vi "DAQ_Dyn Dig Meas Configure and Measure.vi"(0 "DAQmx Task In":refnum<k21>, 2 "Execution Option":T4, 5 "Timing and Trigger Settings":T1={"Timing Settings"={"Sample Clock Source"="OnboardClock", "Sample Rate (Hz)"=10000.0, "Number of Samples"=1000, "Active Edge"=10280}, "Trigger Settings"={"Trigger Type"=enum."No Trigger", "Digital Start Trigger Source"="", "Digital Start Trigger Edge"=10280}} {"Trigger Settings"."Digital Start Trigger Edge" items=["Rising"=10280, "Falling"=10171]; "Timing Settings"."Active Edge" items=["Rising"=10280, "Falling"=10171]; "Timing Settings"."Number of Samples" format="%.0p"; "Timing Settings"."Sample Rate (Hz)" format="%#_6p"}, 11 "error in":errorcluster) -> (4 "DAQmx Task Out":refnum<k21>, 6 "Measured Digital Patterns":digitalwaveform(graph), 8 "Port Digital Data":u32[](array[numeric]), 10 "Acquisition Time (s)":dbl format="%#.2p", 15 "error out":errorcluster)   [LabVIEW 2021, in "DAQ_Dynamic Digital Pattern Measurement.lvlib"]
doc: "Configure, initiate and fetch dynamic digital pattern measurements from the channels configured."
uses:
  DAQ_Dynamic Digital Pattern Measurement.lvlib
  Typedefs/Timing & Trigger Settings.ctl
  Typedefs/Timing Settings.ctl
  Typedefs/Trigger Settings.ctl
  Common/Typedefs/Execution Options - Measure.ctl
  <vilib>/DAQmx/read.llb/DAQmx Read (Digital 1D Wfm NChan NSamp).vi
  <vilib>/DAQmx/configure/timing.llb/DAQmx Timing (Sample Clock).vi
  <vilib>/DAQmx/configure/trigger.llb/DAQmx Start Trigger (Digital Edge).vi
  <vilib>/DAQmx/miscellaneous.llb/DAQmx Fill In Error Info.vi
  <resource>/objmgr/daqmx.rc
panel:
  # "Outputs"
  # "Inputs"
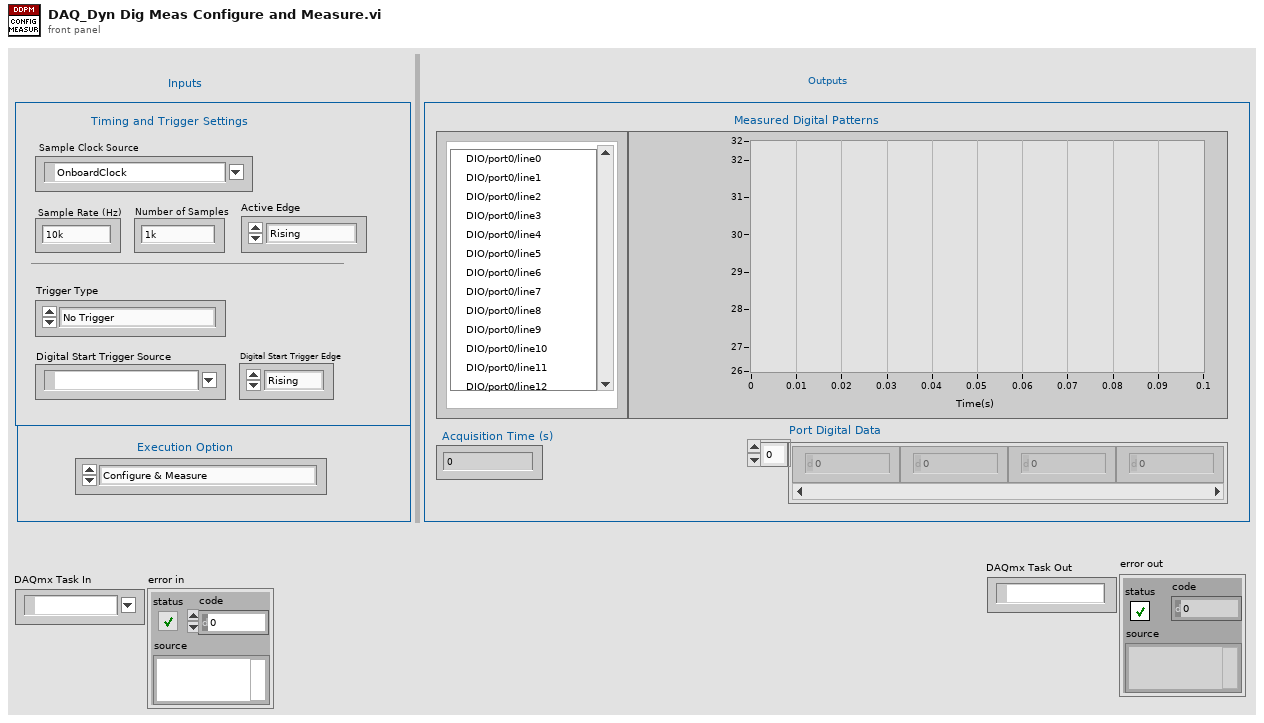
[diagram p1: front panel]
types:
  T1 = typedef "DAQ_Dynamic Digital Pattern Measurement.lvlib/Timing & Trigger Settings.ctl" = cluster{"Timing Settings":T2, "Trigger Settings":T3}
  T2 = typedef "DAQ_Dynamic Digital Pattern Measurement.lvlib/Timing Settings.ctl" = cluster{"Sample Clock Source":tag, "Sample Rate (Hz)":dbl, "Number of Samples":i32, "Active Edge":i32}
  T3 = typedef "DAQ_Dynamic Digital Pattern Measurement.lvlib/Trigger Settings.ctl" = cluster{"Trigger Type":enum16{"No Trigger", "Digital Start"}, "Digital Start Trigger Source":tag, "Digital Start Trigger Edge":i32}
  T4 = typedef "Execution Options - Measure.ctl" = enum16{"Configure & Measure", "Configure only", "Measure only"}
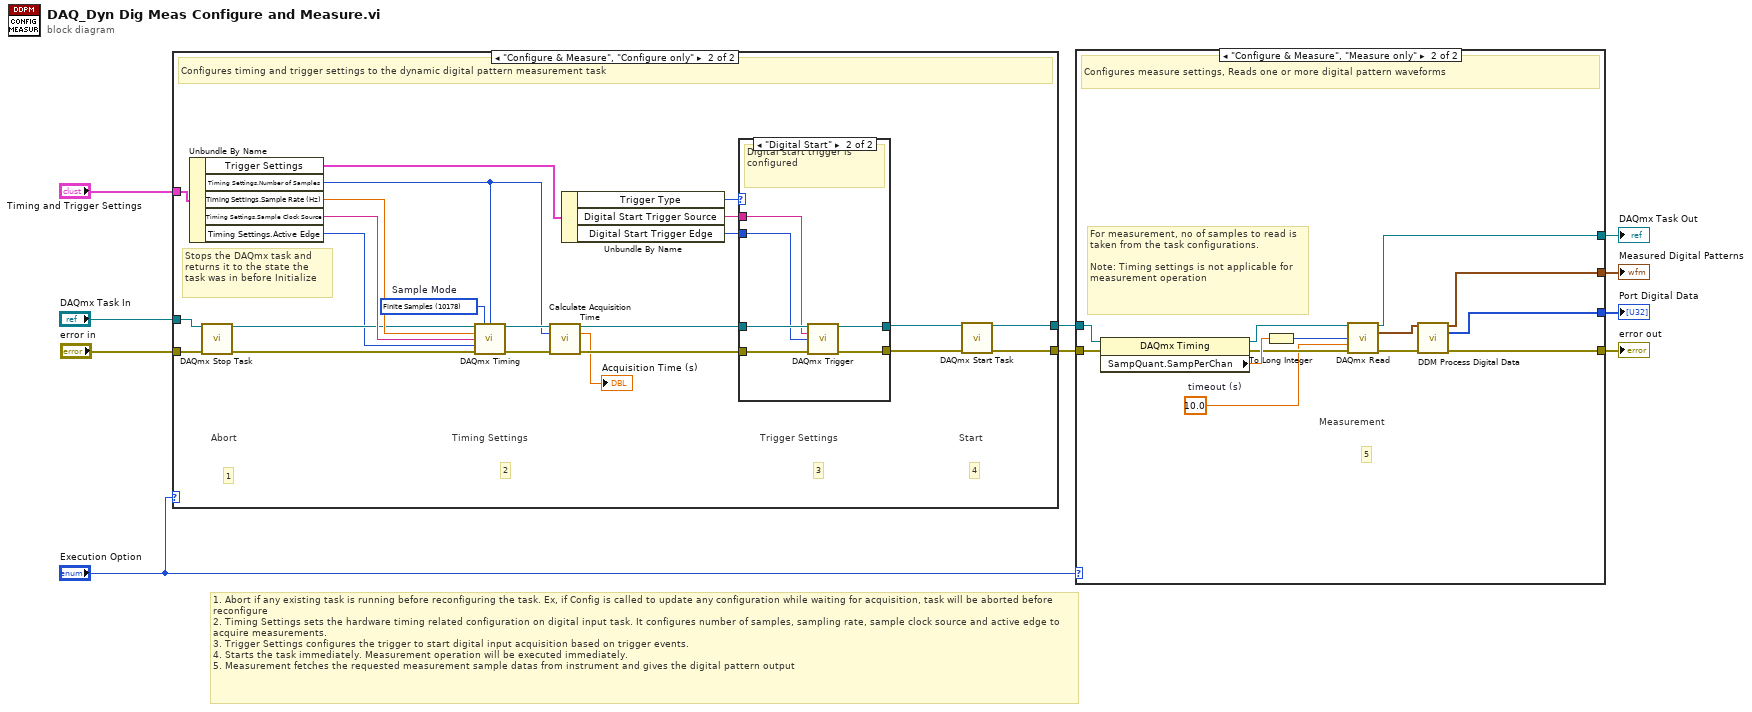
[diagram p0: block diagram]
diagram:
  # "1. Abort if any existing task is running before reconfiguring the task. Ex, if Config is called to update any configuration while waiting for acquisition, task will be aborted before reconfigure\n2. Timing Settings sets the hardware timing related configuration on digital input task. It configures number of samples, sampling rate, sample clock source and active edge to acquire measurements.\n3. Trigger Settings configures the trigger to start digital input acquisition based on trigger events.\n4. Starts the task immediately. Measurement operation will be executed immediately.\n5. Measurement fetches the requested measurement sample datas from instrument and gives the digital pattern output"
  n1 = case shown="\"Configure & Measure\", \"Configure only\"" "Execution Option" {
    tunnel: "error in" -> [w12 w18]
    tunnel: "DAQmx Task In" -> [w11 w20]
    tunnel: "Timing and Trigger Settings" -> [_ w30]
    tunnel: [w11 w16] -> w9
    tunnel: [w12 w27] -> w10
    frame Default {
      # "Skips Configurations (Channel, Timing and Trigger Settings)"
    }
    frame "Configure & Measure", "Configure only" {
      w14 = 10178 items=["Finite Samples"=10178, "Continuous Samples"=10123, "Hardware Timed Single Point"=12522]  # Sample Mode
      # "Stops the DAQmx task and returns it to the state the task was in before Initialize"
      # "4"
      # "Start"
      # "1"
      # "Abort"
      # "3"
      # "2"
      # "Trigger Settings"
      # "Timing Settings"
      # "Configures timing and trigger settings to the dynamic digital pattern measurement task"
      n2 = Unbundle By Name(w30) -> ("Trigger Settings"=w21:T3, "Timing Settings.Number of Samples"=w26:i32, "Timing Settings.Sample Rate (Hz)"=w31:dbl, "Timing Settings.Sample Clock Source"=w32:tag, "Timing Settings.Active Edge"=w13:i32)
      n3 = call <vilib>:"DAQmx Stop Task.vi"("task/channels in"=w20, "error in"=w18) -> ("task out"=w15:refnum<k21>, "error out"=w19:errorcluster)  [unwired: 12 in]
      n4 = call-poly <vilib>:"DAQmx Timing.vi"("task/channels in"=w15, "sample mode"=w14, "samples per channel"=w26, "rate"=w31, "source"=w32, "active edge"=w13, "error in"=w19) -> ("task out"=w35:refnum<k21>, "error out"=w34:errorcluster)  [unwired: 7 in]
      n5 = call "Calculate Acquisition Time.vi"("Refnum in"=w35, "Number of Samples"=w26, "error in (no error)"=w34) -> ("Refnum out"=w28:refnum<k21>, "Acquisition Time Period (s)"=→"Acquisition Time (s)":dbl, "error out"=w33:errorcluster)  [unwired: 10 in]
      n6 = Unbundle By Name(w21) -> ("Trigger Type"=w22:enum16{"No Trigger", "Digital Start"}, "Digital Start Trigger Source"=w24:tag, "Digital Start Trigger Edge"=w23:i32)
      n7 = case shown="\"Digital Start\"" w22 {
        tunnel: w28 -> [w37 w43]
        tunnel: w33 -> [w36 w42]
        tunnel: [w37 w41] -> w17
        tunnel: [w36 w40] -> w29
        tunnel: w24 -> [_ w39]
        tunnel: w23 -> [_ w38]
        frame Default {
          # "No Trigger settings has been configured"
        }
        frame "Digital Start" {
          # "Digital start trigger is configured"
          n8 = call-poly <vilib>:"DAQmx Trigger.vi"("task/channels in"=w43, "source"=w39, "edge"=w38, "error in"=w42) -> ("task out"=w41:refnum<k21>, "error out"=w40:errorcluster)  [unwired: 10 in]
        }
      }
      n9 = call <vilib>:"DAQmx Start Task.vi"("task/channels in"=w17, "error in"=w29) -> ("task out"=w16:refnum<k21>, "error out"=w27:errorcluster)  [unwired: 12 in]
    }
  }
  n10 = case shown="\"Configure & Measure\", \"Measure only\"" "Execution Option" {
    tunnel: w9 -> [w45 w52]
    tunnel: w10 -> [w44 w54]
    tunnel: [w45 w58] -> w8
    tunnel: [w44 w47] -> w5
    tunnel: [_ w49] -> w2
    tunnel: [_ w48] -> w1
    frame Default {
      # "Skips Configurations (Measurement)"
    }
    frame "Configure & Measure", "Measure only" {
      w46 = 10.0  # timeout (s)
      # "For measurement, no of samples to read is taken from the task configurations.\n\nNote: Timing settings is not applicable for measurement operation"
      # "5"
      # "Measurement"
      # "Configures measure settings, Reads one or more digital pattern waveforms"
      n11 = property class="DAQmx Timing"(reference=w52, error in=w54) -> (reference out=w57:refnum<k21>, error out=w55:errorcluster, "SampQuant.SampPerChan"=w56:dbl)
      n12 = To Long Integer(number=w56) -> (32bit integer=w53:i32)
      n13 = call-poly <vilib>:"DAQmx Read.vi"("task/channels in"=w57, "number of samples per channel"=w53, "timeout"=w46, "error in"=w55) -> ("task out"=w58:refnum<k21>, "data"=w50:digitalwaveform[], "error out"=w51:errorcluster)  [unwired: 9 in]
      n14 = call "DDM Process Digital Data.vi"("Captured Digital Waveform In"=w50, "error in (no error)"=w51) -> ("Digital Waveform Out"=w49:digitalwaveform, "Port Digital Data"=w48:u32[], "error out"=w47:errorcluster)  [unwired: 11 in]
    }
  }
  "error out" <- w5
  "DAQmx Task Out" <- w8
  "Port Digital Data" <- w1
  "Measured Digital Patterns" <- w2
